vi "SD_Arduino_Str2Dat.vi"(2 "Arbotix Pin":string="D2", 3 "String from Robot":string="!D0,0,A0,0.17,A1,0.00,A2,0.00,A3,0.00,A4,0.00,A5.0.00,A6,0.00,#") -> (0 "Pin Valid?":bool, 1 "Voltage":dbl)   [LabVIEW 2012]
panel:
  # "Example String from Arbotix Robot"
  # "!D0,0,A0,0.17,A1,0.00,A2,0.00,A3,0.00,A4,0.00,A5.0.00,A6,0.00,#"
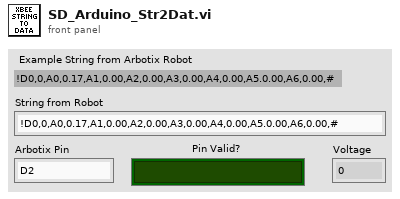
[diagram p1: front panel]
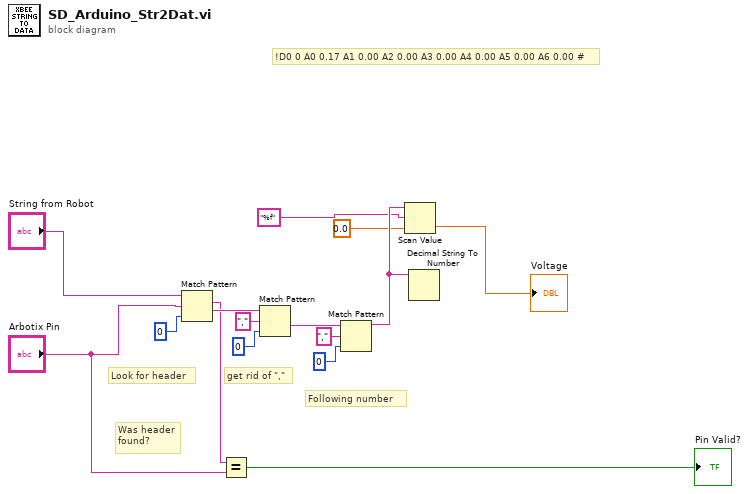
[diagram p0: block diagram]
diagram:
  # "Was header\nfound?"
  # "Following number"
  # "get rid of \",\""
  # "Look for header"
  # "!D0 0 A0 0.17 A1 0.00 A2 0.00 A3 0.00 A4 0.00 A5 0.00 A6 0.00 #"
  n1 = Match Pattern(string="String from Robot", regular expression="Arbotix Pin", offset (0)=0) -> (match substring=w8:string, after substring=w10:string)  [unwired: 2 out]
  n2 = Equal?(x=w8, y="Arbotix Pin") -> (x = y?=→"Pin Valid?":bool)
  n3 = Match Pattern(string=w10, regular expression=",", offset (0)=0) -> (after substring=w11:string)  [unwired: 3 out]
  n4 = Match Pattern(string=w11, regular expression=",", offset (0)=0) -> (before substring=w5:string)  [unwired: 3 out]
  n5 = Scan Value(string=w5, format string="%f", default (0 dbl)=0.0) -> (value=→"Voltage":dbl)  [unwired: 1 out]
  n6 = Decimal String To Number(string=w5) -> ()  [unwired: 2 in, 2 out]
